vi "Periodic Tasks.vi"(8 "error in":errorcluster) -> ()   [LabVIEW 2019]
doc: "This VI runs in parallel to other tasks. It can contain as many user-defined periodic loops as you need. These can carry out PID or other sorts of timed response."
uses:
  <vilib>/Rock Robotics/WPI/DriverStation/WPI_DriverStationRobotMode2.ctl
  LabVIEW_is_Under_Control.lib/Util/Toggle/Change Detect.vi
  LabVIEW_is_Under_Control.lib/Util/Toggle/Change Detect Boolean.vi
  <vilib>/Rock Robotics/WPI/Utilities/WPI_GetSetVariantRefNum.vi
  Robot Global Data.vi
  StateMachine_Global.vi
  Axes_n_Buttons_Global.vi
  Actuators_n_Sensor_Global.vi
  <vilib>/Rock Robotics/WPI/ThirdParty/Phoenix-LabVIEW/Motor Controller/Controls/CTRE_Phoenix_MotorControl_ControlMode.ctl
  <vilib>/Rock Robotics/WPI/Solenoid/WPI_SolenoidValue.ctl
  <vilib>/Rock Robotics/WPI/Solenoid/WPI_SolenoidSetEnum.vi
  <vilib>/Rock Robotics/Network Tables/NT Read Number.vi
  <vilib>/Rock Robotics/Network Tables/NT Write Number.vi
  StateMachines/Turret_Control.ctl
  StateMachines/Climber_Control.ctl
  <vilib>/Rock Robotics/WPI/ThirdParty/Phoenix-LabVIEW/Motor Controller/Controls/CTRE_Phoenix_MotorControl_FeedbackDevice.ctl
  <vilib>/Rock Robotics/WPI/ThirdParty/Phoenix-LabVIEW/Motor Controller/Get/CTRE_Phoenix_MotorController_GetSelectedSensorData.vi
  <vilib>/Rock Robotics/WPI/ThirdParty/Phoenix-LabVIEW/Motor Controller/Get/CTRE_Phoenix_MotorController_GetVoltage.vi
  StateMachines/Ball_Control.ctl
panel:
  in  "Corsair Control":T1(tab)=enum."Turret"
  out "Right Current":dbl
  out "Left Current":dbl
  out "Reversed?":bool
  out "Left Side Current":cluster{"current (A)":dbl, "current (A)":dbl}(graph)
  in  "Sensitivity":dbl=1.5
  out "Right Side Current":cluster{"current (A)":dbl, "current (A)":dbl}(graph)
  out "Voltage Chart":cluster{"Percent Output":dbl}(graph)
  in  "I Zone":dbl
  in  "kF":dbl
  in  "D":dbl
  in  "I":dbl
  in  "P":dbl
  in  "Neutral to Full Seconds":dbl=0.2
  out "Shooter PID Chart":cluster{"Shooter Setpoint":dbl, dbl}(graph)
  out "Voltage Chart Hood":cluster{"Percent Output":dbl}(graph)
  out "Shooter PID Chart Hood":cluster{"Shooter Setpoint":dbl, dbl}(graph)
  in  "I Zone Hood":dbl
  in  "kF Hood":dbl
  in  "D Hood":dbl
  in  "I Hood":dbl
  in  "P Hood":dbl
  in  "Neutral to Full Seconds Hood":dbl=0.2
  out "Turret PID Chart":cluster{"Turret Setpoint":dbl, "TAoutput":dbl}(graph)
  in  "TARange":cluster{"output high":dbl, "output low":dbl}={"output high"=0.6, "output low"=-0.6} {"output low" format="%.2f"; "output high" format="%.2f"}
  in  "TAIntegral Range":dbl=10000.0
  in  "TADisable Range":dbl
  in  "TAGains":T2={"proportional gain (Kc)"=1.0, "integral time (Ti, min)"=0.01, "derivative time (Td, min)"=0.0} {"derivative time (Td, min)" format="%.3f"; "integral time (Ti, min)" format="%.3f"; "proportional gain (Kc)" format="%.3f"}
  out "Hood PID Chart":cluster{"Turret Setpoint":dbl, "TAoutput":dbl}(graph)
  in  "HGains":T2={"proportional gain (Kc)"=1.0, "integral time (Ti, min)"=0.01, "derivative time (Td, min)"=0.0} {"derivative time (Td, min)" format="%.3f"; "integral time (Ti, min)" format="%.3f"; "proportional gain (Kc)" format="%.3f"}
  in  "HDisable Range":dbl
  in  "HIntegral Range":dbl=10000.0
  in  "HRange":cluster{"output high":dbl, "output low":dbl}={"output high"=0.6, "output low"=-0.6} {"output low" format="%.2f"; "output high" format="%.2f"}
  in  "Climber Setpoint":dbl
  in  "Climber Output":dbl
  in  "PDP Port":i32
  out "Current":dbl
  out "Pressing?":bool
  in  "Debug %":dbl
  out "Debug Current":cluster{"current (A)":dbl}(graph)
  # "Press USB 0 A button"
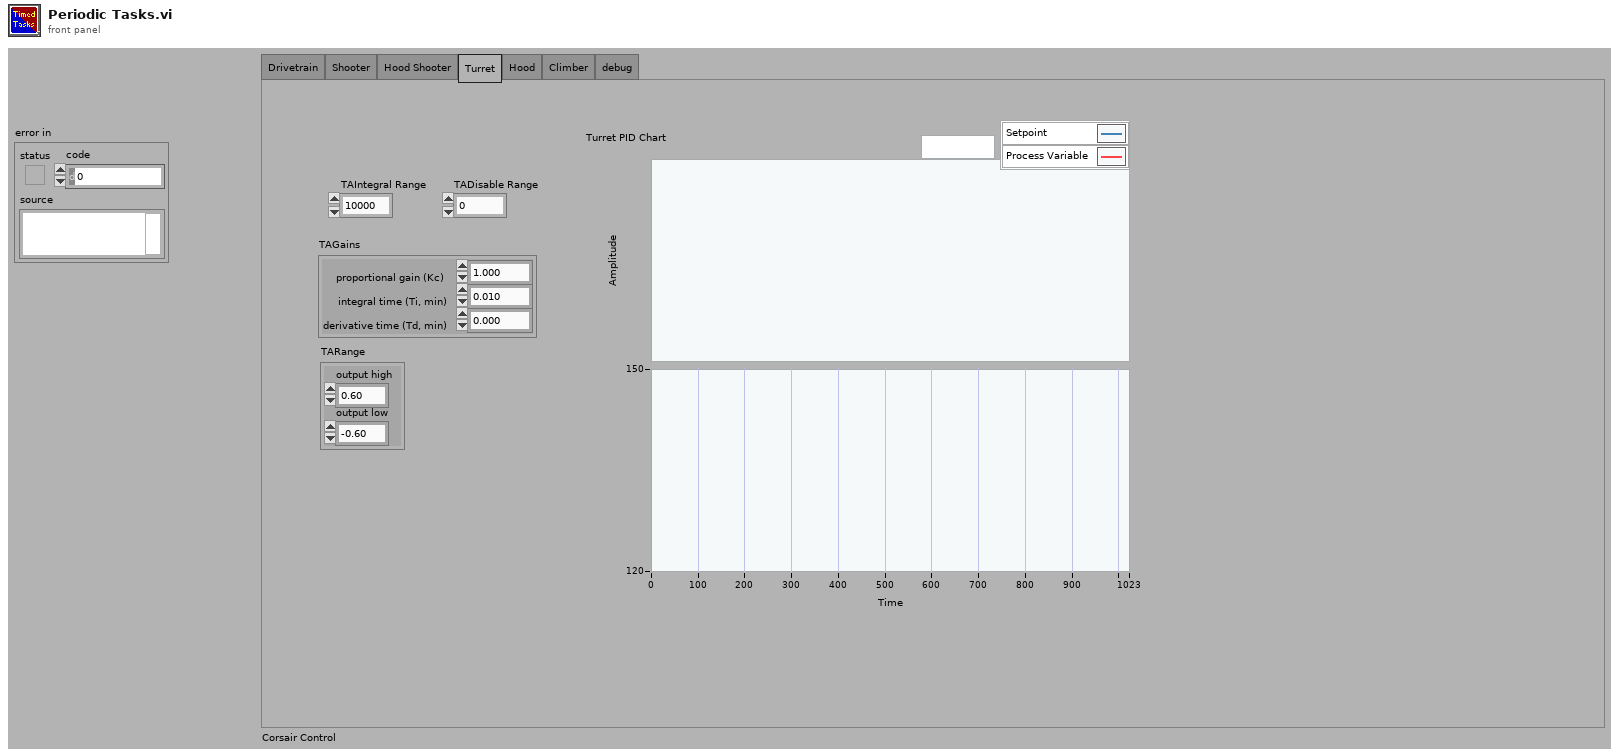
[diagram p1: front panel]
types:
  T1 = enum32{"Drivetrain", "Shooter", "Hood Shooter", "Turret", "Hood", "Climber", "debug"}
  T2 = cluster{"proportional gain (Kc)":dbl, "integral time (Ti, min)":dbl, "derivative time (Td, min)":dbl}
  T3 = typedef "WPI_MotorControlDeviceRef.ctl" = cluster{"DeviceStatus":errorcluster, "Type":T4, "PWM":cluster{"PWM Channel":T5, "DeadBand":T6}, "CAN":cluster{"Device Number":u8, "SetOutput VI Ref":variant, "GetOutput VI Ref":variant, "Enable VI Ref":variant, "Disable VI Ref":variant, "Data":variant}, "Invert":bool, "DIO PWM":cluster{"PWM \"Enable\" Channel":T5, "DIOChannel":T7, "PWM Rate":dbl}}
  T4 = typedef "WPI_MotorControlType.ctl" = enum16{"PWM", "CAN", "DIO PWM"}
  T5 = typedef "FPGA_DIOPWMChannel.ctl" = enum8{"PWM 0", "PWM 1", "PWM 2", "PWM 3", "PWM 4", "PWM 5", "PWM 6", "PWM 7", "PWM 8", "PWM 9", "PWM MXP 0", "PWM MXP 1", "PWM MXP 2", "PWM MXP 3", "PWM MXP 4", "PWM MXP 5", "PWM MXP 6", "PWM MXP 7", "PWM MXP 8", "PWM MXP 9", "Invalid"}
  T6 = typedef "WPI_PWMDeadband.ctl" = cluster{"Name":string, "maxPositivePwm":i32, "minPositivePwm":i32, "centerPwm":i32, "maxNegativePwm":i32, "minNegativePwm":i32, "angularRange":u16}
  T7 = typedef "FPGA_DIOChannel.ctl" = enum8{"DIO 0", "DIO 1", "DIO 2", "DIO 3", "DIO 4", "DIO 5", "DIO 6", "DIO 7", "DIO 8", "DIO 9", "DIO MXP 0", "DIO MXP 1", "DIO MXP 2", "DIO MXP 3", "DIO MXP 4", "DIO MXP 5", "DIO MXP 6", "DIO MXP 7", "DIO MXP 8", "DIO MXP 9", "DIO MXP 10", "DIO MXP 11", "DIO MXP 12", "DIO MXP 13", "DIO MXP 14", "DIO MXP 15", "SPI Port CS1", "SPI Port CS2", "SPI Port CS3", "SPI Port MISO", "SPI Port MOSI", "Invalid"}
  T8 = typedef "WPI_SolenoidDevRef.ctl" = cluster{"DevStatus":errorcluster, "Pneumatics Control Module":u8, "Forward Solenoid Channel":T9, "Reverse Solenoid Channel":T9}
  T9 = typedef "WPI_SolenoidChannel.ctl" = enum8{"Solenoid 0", "Solenoid 1", "Solenoid 2", "Solenoid 3", "Solenoid 4", "Solenoid 5", "Solenoid 6", "Solenoid 7", "Invalid"}
  T10 = typedef "WPI_EncoderDevRef.ctl" = cluster{"DevStatus":errorcluster, "EncoderIndex":T11, "CounterIndex":T12, "DistancePerCount":dbl, "Decoding Type":T13}
  T11 = typedef "FPGA_EncoderIdx.ctl" = enum8{"Enc 0", "Enc 1", "Enc 2", "Enc 3", "Enc 4", "Enc 5", "Enc 6", "Enc 7", "Invalid"}
  T12 = typedef "FPGA_CounterCtrSystemIndex.ctl" = enum8{"Ctr 0", "Ctr 1", "Ctr 2", "Ctr 3", "Ctr 4", "Ctr 5", "Ctr 6", "Ctr 7", "Invalid"}
  T13 = typedef "WPI_EncoderType.ctl" = enum16{"1x", "2x", "4x"}
  T14 = typedef "WPI_RobotDriveDevRef.ctl" = cluster{"DevStatus":errorcluster, "Motors[]":T3[], "Square Inputs":bool, "Max Output":dbl}
  T15 = typedef "WPI_JoystickDevRef.ctl" = cluster{"Device":T16}
  T16 = typedef "WPI_JoystickDeviceEnum.ctl" = enum16{"USB 0", "USB 1", "USB 2", "USB 3", "USB 4", "USB 5"}
  T17 = typedef "WPI_SolenoidValue.ctl" = enum16{"Off", "On", "Forward", "Reverse"}
  T18 = typedef "CTRE_Phoenix_MotorControl_ControlMode.ctl" = u16
  T19 = cluster{"Motors[][0]":T3, "Motors[][1]":T3, "Motors[][2]":T3, "Motors[][3]":T3, "Motors[][4]":T3, "Motors[][5]":T3, "Motors[][6]":T3, "Motors[][7]":T3, "Motors[][8]":T3}
  T20 = typedef "Ball_Control.ctl" = enum16{"Default", "Collect Power Cells", "Prepare Shooter", "Shoot", "Climber Lock"}
  T21 = typedef "Climber_Control.ctl" = enum16{"Locked", "Extend", "Aligned", "Pull", "Lock PTO"}
  T22 = typedef "Turret_Control.ctl" = enum16{"Static", "PreDefined", "Limelight", "Free Control", "Dragoon Mode"}
  T23 = typedef "CTRE_Phoenix_MotorControl_FeedbackDevice.ctl" = i8
  T24 = typedef "WPI_DriverStationRobotMode2.ctl" = enum16{"Autonomous Disabled", "Autonomous Enabled", "Teleop Disabled", "Teleop Enabled", "Disconnected", "Finish", "Test Disabled", "Test Enabled", "Emergency Stopped"}
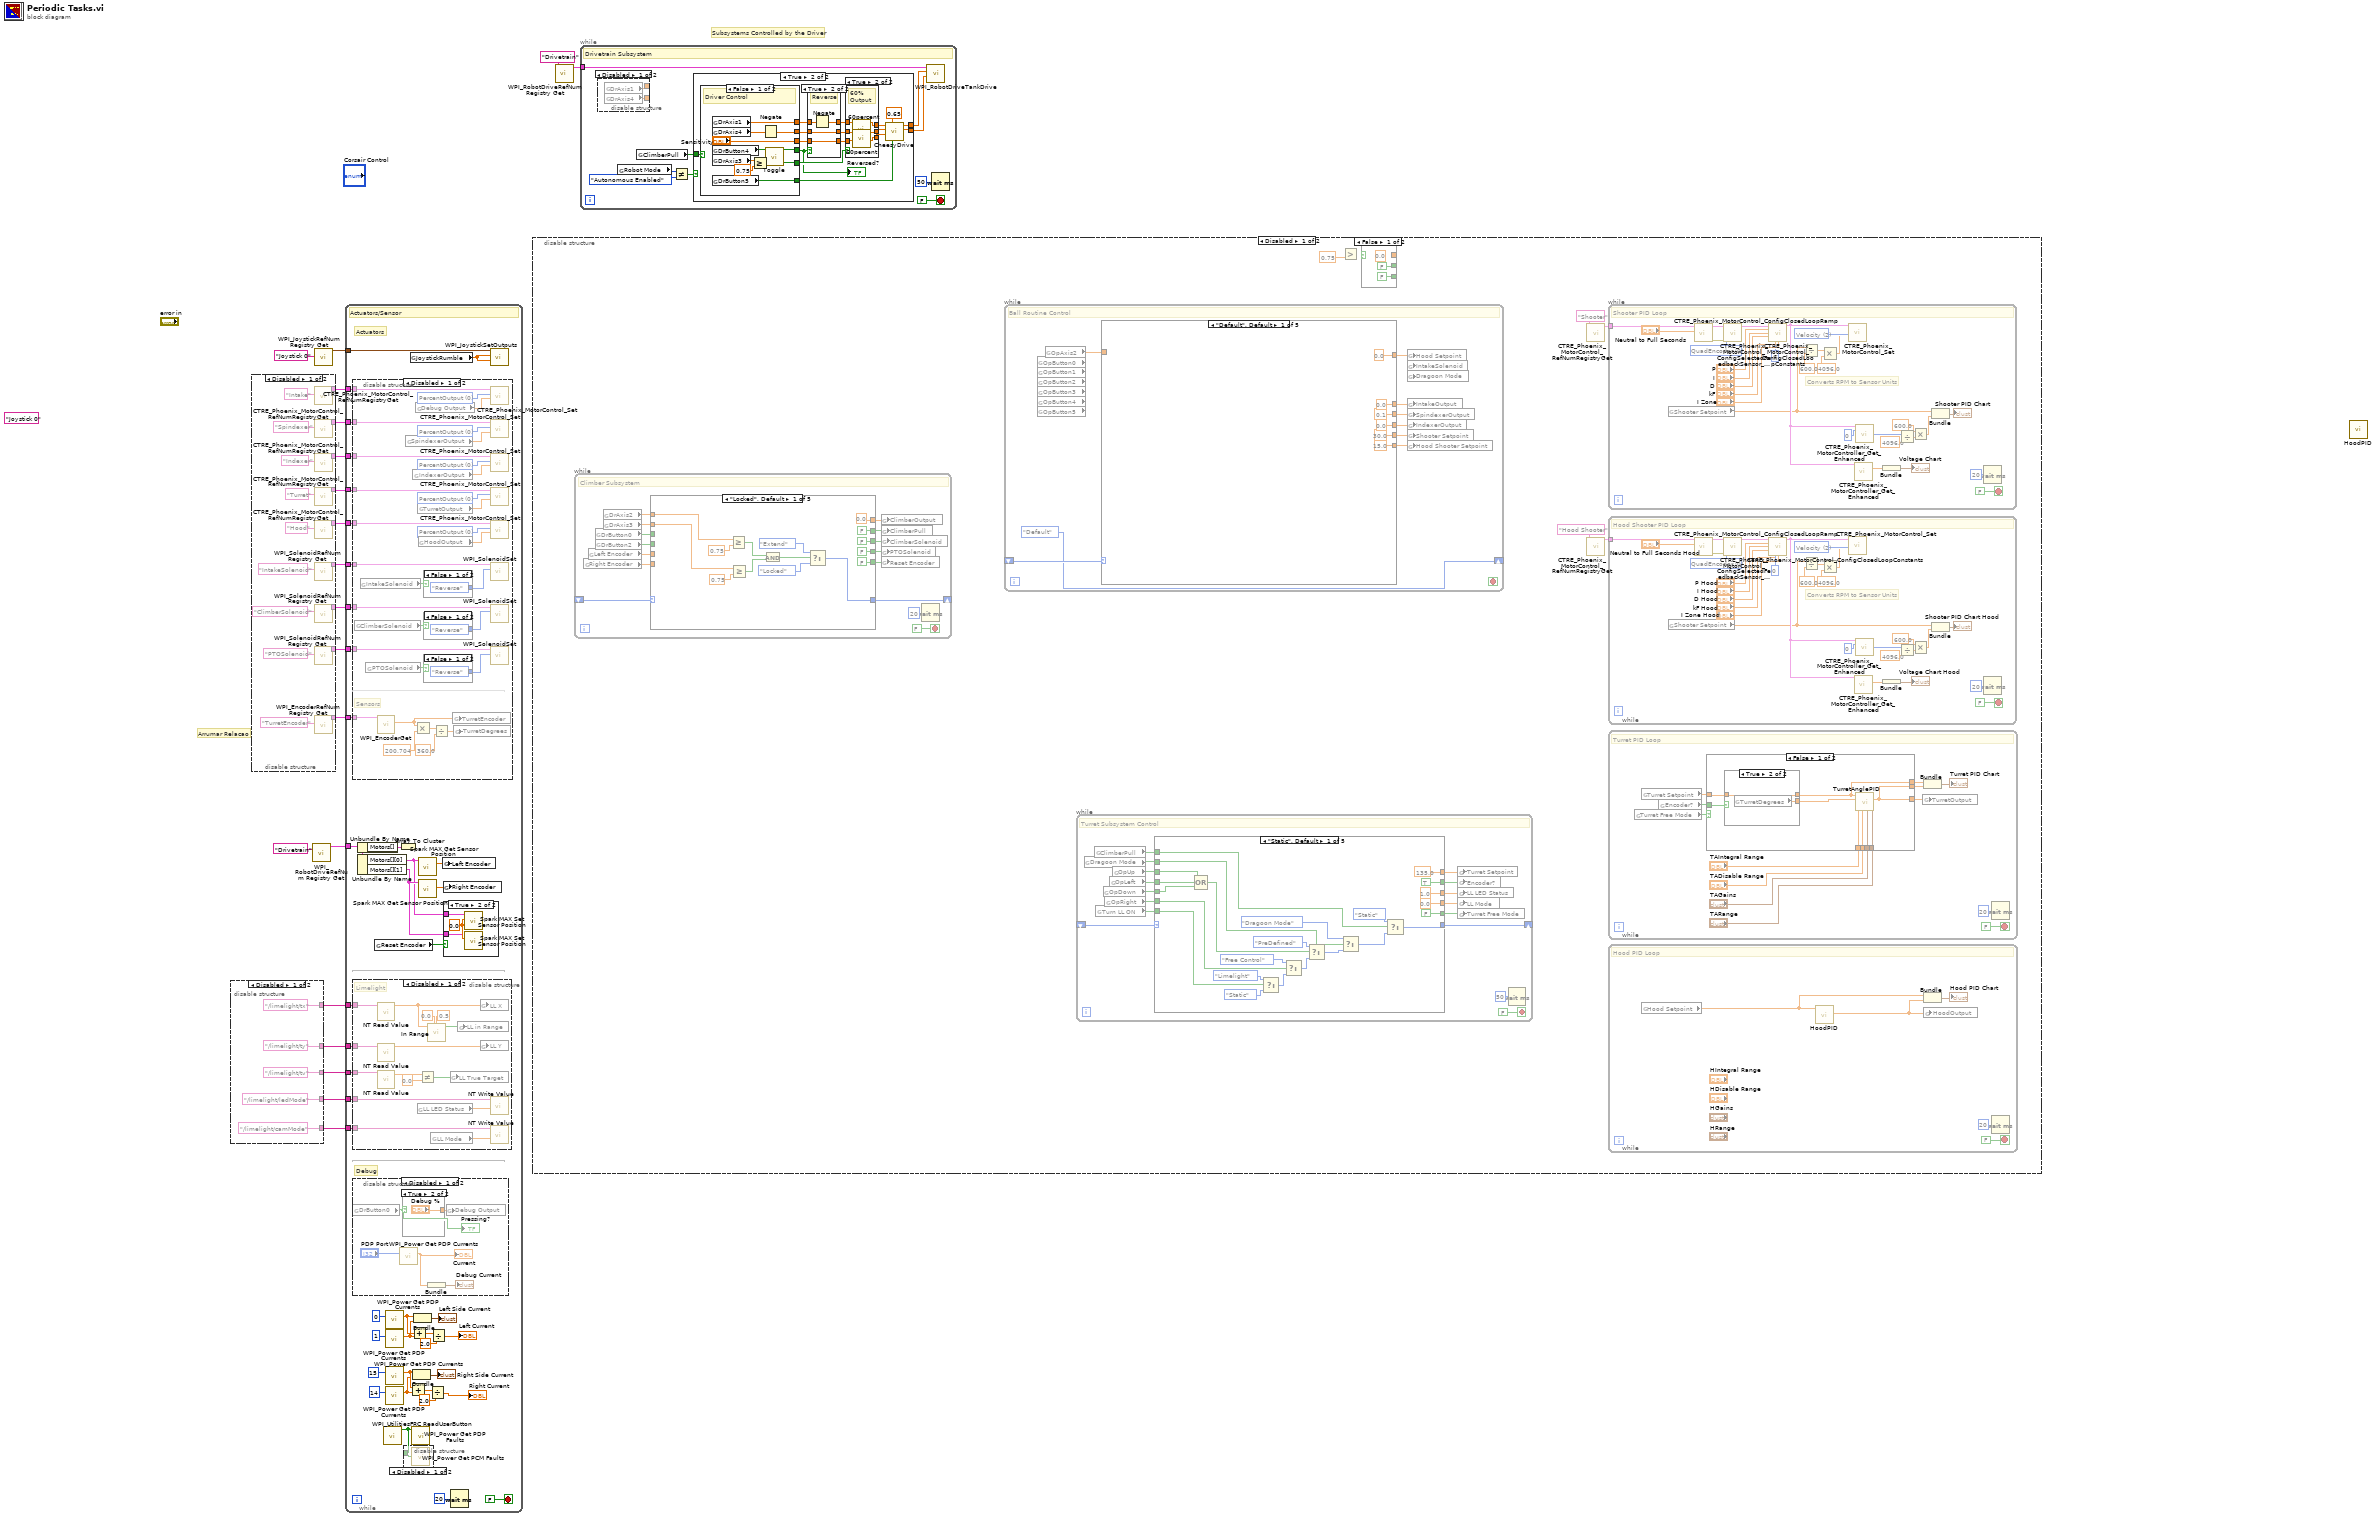
[diagram p0: block diagram]
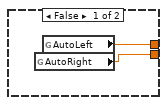
[diagram p3: hidden frame]
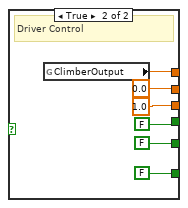
[diagram p5: hidden frame]
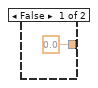
[diagram p9: hidden frame]
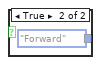
[diagram p13: hidden frame]
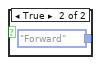
[diagram p14: hidden frame]
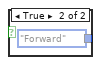
[diagram p15: hidden frame]
diagram:
  (unwired) "Joystick 0" ("refnum name")
  # "Subsystems Controlled by the Driver"
  # "Arrumar Relacao"
  n1 = disable-structure shown="Disabled" {
    disable-tunnel: ["/limelight/tx" ("Name") _] -> w13
    disable-tunnel: ["/limelight/ty" ("Name") _] -> w12
    disable-tunnel: ["/limelight/tv" ("Name") _] -> w11
    disable-tunnel: ["/limelight/ledMode" ("Name") _] -> w10
    disable-tunnel: ["/limelight/camMode" ("Name") _] -> w9
    frame Disabled {
    }
    frame Enabled {
    }
  }
  n2 = disable-structure shown="Disabled" {
    disable-tunnel: [w42 _] -> w20
    disable-tunnel: [w41 _] -> w19
    disable-tunnel: [w38 _] -> w18
    disable-tunnel: [w37 _] -> w17
    disable-tunnel: [w34 _] -> w16
    disable-tunnel: [w33 _] -> w15
    disable-tunnel: [w32 _] -> w7
    disable-tunnel: [w31 _] -> w6
    disable-tunnel: [w30 _] -> w5
    frame Disabled {
      n3 = call <vilib>:"CTRE_Phoenix_MotorControl_RefNumRegistryGet.vi"("refnum name"="Intake") -> ("PhoenixMotorControlDevRef"=w42:T3)  [unwired: 9 in, 1 out]
      n4 = call <vilib>:"CTRE_Phoenix_MotorControl_RefNumRegistryGet.vi"("refnum name"="Spindexer") -> ("PhoenixMotorControlDevRef"=w41:T3)  [unwired: 9 in, 1 out]
      n5 = call <vilib>:"CTRE_Phoenix_MotorControl_RefNumRegistryGet.vi"("refnum name"="Indexer") -> ("PhoenixMotorControlDevRef"=w38:T3)  [unwired: 9 in, 1 out]
      n6 = call <vilib>:"CTRE_Phoenix_MotorControl_RefNumRegistryGet.vi"("refnum name"="Turret") -> ("PhoenixMotorControlDevRef"=w37:T3)  [unwired: 9 in, 1 out]
      n7 = call <vilib>:"CTRE_Phoenix_MotorControl_RefNumRegistryGet.vi"("refnum name"="Hood") -> ("PhoenixMotorControlDevRef"=w34:T3)  [unwired: 9 in, 1 out]
      n8 = call <vilib>:"WPI_SolenoidRefNum Registry Get.vi"("refnum name"="IntakeSolenoid") -> ("SolenoidDevRef"=w32:T8)  [unwired: 9 in, 1 out]
      n9 = call <vilib>:"WPI_SolenoidRefNum Registry Get.vi"("refnum name"="ClimberSolenoid") -> ("SolenoidDevRef"=w31:T8)  [unwired: 9 in, 1 out]
      n10 = call <vilib>:"WPI_SolenoidRefNum Registry Get.vi"("refnum name"="PTOSolenoid") -> ("SolenoidDevRef"=w30:T8)  [unwired: 9 in, 1 out]
      n11 = call <vilib>:"WPI_EncoderRefNum Registry Get.vi"("refnum name"="TurretEncoder") -> ("EncoderDevRef"=w33:T10)  [unwired: 9 in, 1 out]
    }
    frame Enabled {
    }
  }
  n12 = call <vilib>:"WPI_RobotDriveRefNum Registry Get.vi"("refnum name"="Drivetrain") -> ("RobotDriveDevRef"=w3:T14)  [unwired: 9 in, 1 out]
  n13 = call <vilib>:"WPI_JoystickRefNum Registry Get.vi"("refnum name"="Joystick 0") -> ("JoystickDevRef"=w14:T15)  [unwired: 9 in, 1 out]
  n14 = while {
    tunnel: w20 -> [w86]
    tunnel: w19 -> [w85]
    tunnel: w18 -> [w84]
    tunnel: w17 -> [w83]
    tunnel: w16 -> [w82]
    tunnel: w15 -> [w81]
    tunnel: w14 -> [w80]
    tunnel: w13 -> [w78]
    tunnel: w12 -> [w77]
    tunnel: w11 -> [w76]
    tunnel: w10 -> [w75]
    tunnel: w9 -> [w74]
    tunnel: w7 -> [w72]
    tunnel: w6 -> [w71]
    tunnel: w5 -> [w70]
    tunnel: w3 -> [w69]
    stop <- FALSE stop-if-true
    # "Debug"
    # "Actuators"
    # "Actuators/Sensor"
    n15 = disable-structure shown="Disabled" {
      disable-tunnel: w86 -> [w139 _]
      disable-tunnel: w85 -> [w138 _]
      disable-tunnel: w84 -> [w137 _]
      disable-tunnel: w83 -> [w136 _]
      disable-tunnel: w82 -> [w135 _]
      disable-tunnel: w81 -> [w128 _]
      disable-tunnel: w72 -> [w117 _]
      disable-tunnel: w71 -> [w116 _]
      disable-tunnel: w70 -> [w115 _]
      frame Disabled {
        w126 = T18 0 items=["PercentOutput"=0, "Position"=1, "Velocity"=2, "Current"=3, "Follower"=5, "MotionProfile"=6, "MotionMagic"=7, "MotionProfileArc"=10, "Disabled"=15] ("Control Mode")
        w121 = T18 0 items=["PercentOutput"=0, "Position"=1, "Velocity"=2, "Current"=3, "Follower"=5, "MotionProfile"=6, "MotionMagic"=7, "MotionProfileArc"=10, "Disabled"=15] ("Control Mode")
        w123 = T18 0 items=["PercentOutput"=0, "Position"=1, "Velocity"=2, "Current"=3, "Follower"=5, "MotionProfile"=6, "MotionMagic"=7, "MotionProfileArc"=10, "Disabled"=15] ("Control Mode")
        w125 = T18 0 items=["PercentOutput"=0, "Position"=1, "Velocity"=2, "Current"=3, "Follower"=5, "MotionProfile"=6, "MotionMagic"=7, "MotionProfileArc"=10, "Disabled"=15] ("Control Mode")
        w127 = T18 0 items=["PercentOutput"=0, "Position"=1, "Velocity"=2, "Current"=3, "Follower"=5, "MotionProfile"=6, "MotionMagic"=7, "MotionProfileArc"=10, "Disabled"=15] ("Control Mode")
        # "Sensors"
        n16 = global read "Actuators_n_Sensor_Global.vi" "ClimberSolenoid"() -> (w132:bool)
        n17 = global read "Actuators_n_Sensor_Global.vi" "IntakeSolenoid"() -> (w133:bool)
        n18 = global read "Actuators_n_Sensor_Global.vi" "PTOSolenoid"() -> (w129:bool)
        n19 = call <vilib>:"WPI_EncoderGet.vi"("EncoderDevRef"=w128) -> ("Distance"=w110:dbl)  [unwired: 5 in, 5 out]
        n20 = global read "Actuators_n_Sensor_Global.vi" "SpindexerOutput"() -> (w124:dbl)
        n21 = global read "Actuators_n_Sensor_Global.vi" "IndexerOutput"() -> (w122:dbl)
        n22 = Multiply(x=w110, y=200.704) -> (x*y=w113:dbl)
        n23 = global read "Actuators_n_Sensor_Global.vi" "Debug Output"() -> (w118:dbl)
        n24 = global read "Actuators_n_Sensor_Global.vi" "TurretOutput"() -> (w120:dbl)
        n25 = global read "Actuators_n_Sensor_Global.vi" "HoodOutput"() -> (w119:dbl)
        n26 = case shown="False" w133 {
          tunnel: [WPI_SolenoidValue."Reverse" ("Value") WPI_SolenoidValue."Forward" ("Value")] -> w134
          frame False {
          }
          frame True {
          }
        }
        n27 = case shown="False" w132 {
          tunnel: [WPI_SolenoidValue."Reverse" ("Value") WPI_SolenoidValue."Forward" ("Value")] -> w131
          frame False {
          }
          frame True {
          }
        }
        n28 = case shown="False" w129 {
          tunnel: [WPI_SolenoidValue."Reverse" ("Value") WPI_SolenoidValue."Forward" ("Value")] -> w130
          frame False {
          }
          frame True {
          }
        }
        n29 = Divide(x=w113, y=360.0) -> (x/y=w111:dbl)
        n30 = global write "Actuators_n_Sensor_Global.vi" "TurretEncoder"(w110) -> ()
        n31 = global write "Actuators_n_Sensor_Global.vi" "TurretDegrees"(w111) -> ()
        n32 = call <vilib>:"CTRE_Phoenix_MotorControl_Set.vi"("Output"=w118, "Control Mode"=w127, "PhoenixMotorControlDevRef"=w139) -> ()  [unwired: 7 in, 2 out]
        n33 = call <vilib>:"CTRE_Phoenix_MotorControl_Set.vi"("Output"=w124, "Control Mode"=w125, "PhoenixMotorControlDevRef"=w138) -> ()  [unwired: 7 in, 2 out]
        n34 = call <vilib>:"CTRE_Phoenix_MotorControl_Set.vi"("Output"=w122, "Control Mode"=w123, "PhoenixMotorControlDevRef"=w137) -> ()  [unwired: 7 in, 2 out]
        n35 = call <vilib>:"CTRE_Phoenix_MotorControl_Set.vi"("Output"=w120, "Control Mode"=w121, "PhoenixMotorControlDevRef"=w136) -> ()  [unwired: 7 in, 2 out]
        n36 = call <vilib>:"CTRE_Phoenix_MotorControl_Set.vi"("Output"=w119, "Control Mode"=w126, "PhoenixMotorControlDevRef"=w135) -> ()  [unwired: 7 in, 2 out]
        n37 = call-poly <vilib>:"WPI_SolenoidSet.vi"("Value"=w134, "SolenoidDevRef"=w117) -> ()  [unwired: 8 in, 2 out]
        n38 = call-poly <vilib>:"WPI_SolenoidSet.vi"("Value"=w131, "SolenoidDevRef"=w116) -> ()  [unwired: 8 in, 2 out]
        n39 = call-poly <vilib>:"WPI_SolenoidSet.vi"("Value"=w130, "SolenoidDevRef"=w115) -> ()  [unwired: 8 in, 2 out]
      }
      frame Enabled {
      }
    }
    n40 = disable-structure shown="Disabled" {
      frame Disabled {
        n41 = global read "Axes_n_Buttons_Global.vi" "DrButton0"() -> (w88:bool)
        "Pressing?" <- w88
        n42 = call <vilib>:"WPI_Power Get PDP Currents.vi"("PDP Channel"="PDP Port") -> ("current (A)"=w87:dbl)  [unwired: 12 in, 2 out]
        "Current" <- w87
        n43 = case shown="True" w88 {
          tunnel: [0.0 ("Test") "Debug %"] -> w91
          frame False {
          }
          frame True {
          }
        }
        n44 = Bundle("current (A)"=w87) -> (→"Debug Current":cluster{"current (A)":dbl})  [unwired: 1 in]
        n45 = global write "Actuators_n_Sensor_Global.vi" "Debug Output"(w91) -> ()
      }
      frame Enabled {
      }
    }
    n46 = disable-structure shown="Disabled" {
      disable-tunnel: w78 -> [w101 _]
      disable-tunnel: w77 -> [w100 _]
      disable-tunnel: w76 -> [w99 _]
      disable-tunnel: w75 -> [w98 _]
      disable-tunnel: w74 -> [w97 _]
      frame Disabled {
        # "Limelight"
        n47 = call-poly <vilib>:"NT Read Value.vi"("Name"=w101) -> ("Numeric"=w108:dbl)  [unwired: 9 in, 1 out]
        n48 = call-poly <vilib>:"NT Read Value.vi"("Name"=w100) -> ("Numeric"=w105:dbl)  [unwired: 9 in, 1 out]
        n49 = call-poly <vilib>:"NT Read Value.vi"("Name"=w99) -> ("Numeric"=w103:dbl)  [unwired: 9 in, 1 out]
        n50 = global read "Actuators_n_Sensor_Global.vi" "LL LED Status"() -> (w96:dbl)
        n51 = Not Equal?(x=w103, y=0.0) -> (x != y?=w102:bool)
        n52 = call "In Range.vi"("Range"=0.5, "Setpoint"=0.0, "Value"=w108) -> ("in range?"=w109:bool)  [unwired: 8 in]
        n53 = global read "Actuators_n_Sensor_Global.vi" "LL Mode"() -> (w95:dbl)
        n54 = global write "Actuators_n_Sensor_Global.vi" "LL True Target"(w102) -> ()
        n55 = global write "Actuators_n_Sensor_Global.vi" "LL in Range"(w109) -> ()
        n56 = global write "Actuators_n_Sensor_Global.vi" "LL X"(w108) -> ()
        n57 = global write "Actuators_n_Sensor_Global.vi" "LL Y"(w105) -> ()
        n58 = call-poly <vilib>:"NT Write Value.vi"("Numeric"=w96, "Name"=w98) -> ()  [unwired: 9 in, 1 out]
        n59 = call-poly <vilib>:"NT Write Value.vi"("Numeric"=w95, "Name"=w97) -> ()  [unwired: 9 in, 1 out]
      }
      frame Enabled {
      }
    }
    n60 = Unbundle By Name(w69) -> ("Motors[]"=w68:T3[])
    n61 = global read "Actuators_n_Sensor_Global.vi" "Reset Encoder"() -> (w64:bool)
    n62 = call <vilib>:"WPI_UtilitiesFRC ReadUserButton.vi"() -> ("User Button"=w60:bool)  [unwired: 10 in, 1 out]
    n63 = call <vilib>:"WPI_Power Get PDP Currents.vi"("PDP Channel"=0) -> ("current (A)"=w53:dbl)  [unwired: 12 in, 2 out]
    n64 = call <vilib>:"WPI_Power Get PDP Currents.vi"("PDP Channel"=1) -> ("current (A)"=w52:dbl)  [unwired: 12 in, 2 out]
    n65 = call <vilib>:"WPI_Power Get PDP Currents.vi"("PDP Channel"=15) -> ("current (A)"=w46:dbl)  [unwired: 12 in, 2 out]
    n66 = call <vilib>:"WPI_Power Get PDP Currents.vi"("PDP Channel"=14) -> ("current (A)"=w45:dbl)  [unwired: 12 in, 2 out]
    n67 = Array To Cluster(array=w68) -> (cluster=w67:T19)
    n68 = Unbundle By Name(w67) -> ("Motors[][0]"=w62:T3, "Motors[][1]"=w63:T3)
    n69 = disable-structure shown="Disabled" {
      disable-tunnel: w60 -> [w94 _]
      frame Disabled {
        n70 = call <vilib>:"WPI_Power Get PCM Faults.vi"("Clear Sticky Faults"=w94) -> ()  [unwired: 11 in, 4 out]
      }
      frame Enabled {
      }
    }
    n71 = Add(x=w46, y=w45) -> (x+y=w47:dbl)
    n72 = global read "Actuators_n_Sensor_Global.vi" "JoystickRumble"() -> (w79:dbl)
    n73 = Add(x=w53, y=w52) -> (x+y=w51:dbl)
    n74 = call <vilib>:"WPI_Power Get PDP Faults.vi"("Clear Sticky Faults"=w60) -> ()  [unwired: 10 in, 5 out]
    n75 = Bundle("current (A)"=w46, "current (A)"=w45) -> (→"Right Side Current":cluster{"current (A)":dbl, "current (A)":dbl})  [unwired: 1 in]
    n76 = Bundle("current (A)"=w53, "current (A)"=w52) -> (→"Left Side Current":cluster{"current (A)":dbl, "current (A)":dbl})  [unwired: 1 in]
    n77 = call <vilib>:"Spark MAX Get Sensor Position.vi"("MotorControlDevRef in"=w62) -> ("Sensor Position"=w66:dbl)  [unwired: 7 in, 3 out]
    n78 = call <vilib>:"Spark MAX Get Sensor Position.vi"("MotorControlDevRef in"=w63) -> ("Sensor Position"=w65:dbl)  [unwired: 7 in, 3 out]
    n79 = Divide(x=w47, y=2.0) -> (x/y=→"Right Current":dbl)
    n80 = Divide(x=w51, y=2.0) -> (x/y=→"Left Current":dbl)
    n81 = global write "Actuators_n_Sensor_Global.vi" "Left Encoder"(w66) -> ()
    n82 = global write "Actuators_n_Sensor_Global.vi" "Right Encoder"(w65) -> ()
    n83 = case shown="True" w64 {
      tunnel: w63 -> [_ w147]
      tunnel: w62 -> [_ w146]
      frame False {
      }
      frame True {
        w148 = 0.0 ("Position")
        n84 = call <vilib>:"Spark MAX Set Sensor Position.vi"("Position"=w148, "MotorControlDeviceRef"=w146) -> ()  [unwired: 8 in, 2 out]
        n85 = call <vilib>:"Spark MAX Set Sensor Position.vi"("Position"=w148, "MotorControlDeviceRef"=w147) -> ()  [unwired: 8 in, 2 out]
      }
    }
    n86 = Wait (ms)(milliseconds to wait=u32 20) -> ()  [unwired: 1 out]
    n87 = call <vilib>:"WPI_JoystickSetOutputs.vi"("Right Rumble"=w79, "Left Rumble"=w79, "JoystickDevRef"=w80) -> ()  [unwired: 7 in, 2 out]
  }
  n88 = disable-structure shown="Disabled" {
    frame Disabled {
      n89 = while {
        shift-right: [w245] -> _
        shift-left: _ -> [w246]
        stop <- FALSE stop-if-true
        # "Climber Subsystem"
        n90 = global read "Actuators_n_Sensor_Global.vi" "Right Encoder"() -> (w239:dbl)
        n91 = global read "Actuators_n_Sensor_Global.vi" "Left Encoder"() -> (w240:dbl)
        n92 = global read "Axes_n_Buttons_Global.vi" "DrButton0"() -> (w242:bool)
        n93 = global read "Axes_n_Buttons_Global.vi" "DrButton2"() -> (w241:bool)
        n94 = global read "Axes_n_Buttons_Global.vi" "DrAxis2"() -> (w244:dbl)
        n95 = global read "Axes_n_Buttons_Global.vi" "DrAxis3"() -> (w243:dbl)
        n96 = case shown="\"Locked\", Default" w246 {
          tunnel: [w257 w265 Climber_Control."Pull" w282 Climber_Control."Lock PTO"] -> w245
          tunnel: w244 -> [w255 _ _ _ _]
          tunnel: w243 -> [w254 _ _ _ _]
          tunnel: w242 -> [_ w266 _ _ _]
          tunnel: w241 -> [_ _ _ _ _]
          tunnel: w240 -> [_ _ _ w292 _]
          tunnel: w239 -> [_ _ _ w293 _]
          tunnel: [FALSE FALSE FALSE TRUE FALSE] -> w238
          tunnel: [0.0 0.0 0.0 "Climber Output" 0.0 ("Climber Output")] -> w237
          tunnel: [FALSE TRUE TRUE TRUE TRUE] -> w236
          tunnel: [FALSE FALSE TRUE TRUE FALSE] -> w235
          tunnel: [FALSE FALSE TRUE FALSE TRUE] -> w234
          frame "Locked", Default {
            n97 = Greater Or Equal?(x=w255, y=0.75) -> (x >= y?=w261:bool)
            n98 = Greater Or Equal?(x=w254, y=0.75) -> (x >= y?=w260:bool)
            n99 = And(x=w261, y=w260) -> (x .and. y?=w259:bool)
            n100 = Select(t=Climber_Control."Extend", s=w259, f=Climber_Control."Locked") -> (s? t:f=w257:T21)
          }
          frame "Extend" {
            n101 = Select(t=Climber_Control."Aligned", s=w266, f=Climber_Control."Extend") -> (s? t:f=w265:T21)
          }
          frame "Aligned" {
          }
          frame "Pull" {
            n102 = Add(x=w292, y=w293) -> (x+y=w291:dbl)
            n103 = Divide(x=w291, y=2.0) -> (x/y=w289:dbl)
            n104 = Greater Or Equal?(x=w289, y="Climber Setpoint") -> (x >= y?=w283:bool)
            n105 = Select(t=Climber_Control."Lock PTO", s=w283, f=Climber_Control."Pull") -> (s? t:f=w282:T21)
          }
          frame "Lock PTO" {
          }
        }
        n106 = global write "StateMachine_Global.vi" "ClimberOutput"(w237) -> ()
        n107 = global write "StateMachine_Global.vi" "ClimberPull"(w238) -> ()
        n108 = global write "Actuators_n_Sensor_Global.vi" "ClimberSolenoid"(w236) -> ()
        n109 = global write "Actuators_n_Sensor_Global.vi" "PTOSolenoid"(w235) -> ()
        n110 = global write "Actuators_n_Sensor_Global.vi" "Reset Encoder"(w234) -> ()
        n111 = Wait (ms)(milliseconds to wait=u32 20) -> ()  [unwired: 1 out]
      }
      n112 = while {
        shift-right: [Ball_Control."Default"] -> _
        shift-left: _ -> [w167]
        stop <- _ stop-if-true
        # "Ball Routine Control"
        n113 = global read "Axes_n_Buttons_Global.vi" "OpButton0"() -> ()  [unwired: 1 out]
        n114 = global read "Axes_n_Buttons_Global.vi" "OpButton1"() -> ()  [unwired: 1 out]
        n115 = global read "Axes_n_Buttons_Global.vi" "OpButton2"() -> ()  [unwired: 1 out]
        n116 = global read "Axes_n_Buttons_Global.vi" "OpButton3"() -> ()  [unwired: 1 out]
        n117 = global read "Axes_n_Buttons_Global.vi" "OpButton4"() -> ()  [unwired: 1 out]
        n118 = global read "Axes_n_Buttons_Global.vi" "OpButton5"() -> ()  [unwired: 1 out]
        n119 = global read "Axes_n_Buttons_Global.vi" "OpAxis2"() -> (w160:dbl)
        n120 = case shown="\"Default\", Default" w167 {
          tunnel: [0.0 _ _ _ _] -> w165
          tunnel: [0.1 _ _ _ _] -> w164
          tunnel: [0.0 _ _ _ _] -> w163
          tunnel: [30.0 _ _ _ _] -> w162
          tunnel: [15.0 _ _ _ _] -> w161
          tunnel: w160 -> [_ _ _ _ _]
          tunnel: [0.0 _ _ _ _] -> w159
          frame "Default", Default {
          }
          frame "Collect Power Cells" {
          }
          frame "Prepare Shooter" {
          }
          frame "Shoot" {
          }
          frame "Climber Lock" {
          }
        }
        n121 = global write "StateMachine_Global.vi" "Hood Setpoint"(w159) -> ()
        n122 = global read "Actuators_n_Sensor_Global.vi" "IntakeSolenoid"() -> ()  [unwired: 1 in]
        n123 = global read "StateMachine_Global.vi" "Dragoon Mode"() -> ()  [unwired: 1 in]
        n124 = global write "Actuators_n_Sensor_Global.vi" "IntakeOutput"(w165) -> ()
        n125 = global write "Actuators_n_Sensor_Global.vi" "SpindexerOutput"(w164) -> ()
        n126 = global write "Actuators_n_Sensor_Global.vi" "IndexerOutput"(w163) -> ()
        n127 = global write "StateMachine_Global.vi" "Shooter Setpoint"(w162) -> ()
        n128 = global write "StateMachine_Global.vi" "Hood Shooter Setpoint"(w161) -> ()
      }
      n129 = while {
        shift-right: [w307] -> _
        shift-left: _ -> [w314]
        stop <- FALSE stop-if-true
        # "Turret Subsystem Control"
        n130 = global read "StateMachine_Global.vi" "Dragoon Mode"() -> (w303:bool)
        n131 = global read "StateMachine_Global.vi" "ClimberPull"() -> (w300:bool)
        n132 = global read "StateMachine_Global.vi" "Turn LL ON"() -> (w308:bool)
        n133 = global read "Axes_n_Buttons_Global.vi" "OpDown"() -> (w310:bool)
        n134 = global read "Axes_n_Buttons_Global.vi" "OpRight"() -> (w309:bool)
        n135 = global read "Axes_n_Buttons_Global.vi" "OpLeft"() -> (w311:bool)
        n136 = global read "Axes_n_Buttons_Global.vi" "OpUp"() -> (w312:bool)
        n137 = case shown="\"Static\", Default" w314 {
          tunnel: [135.0 w344 0.0 ("f") 0.0 ("f") 225.0 ("f")] -> w313
          tunnel: w312 -> [w338 w346 _ _ _]
          tunnel: w311 -> [w337 w347 _ _ _]
          tunnel: w310 -> [w336 w345 _ _ _]
          tunnel: w309 -> [w330 _ _ w364 _]
          tunnel: w308 -> [w329 _ w355 _ _]
          tunnel: [w319 w340 w356 w365 w375] -> w307
          tunnel: [0.0 _ _ _ _] -> w306
          tunnel: [1.0 1.0 0.0 1.0 1.0] -> w305
          tunnel: [TRUE TRUE FALSE FALSE TRUE] -> w304
          tunnel: w303 -> [w322 _ _ _ w374]
          tunnel: [FALSE _ _ TRUE _] -> w302
          tunnel: w300 -> [w316 _ _ _ _]
          frame "Static", Default {
            n138 = Compound Arithmetic op=OR(w338, w337, w336) -> (w335:bool)
            n139 = Select(t=Turret_Control."Limelight", s=w329, f=Turret_Control."Static") -> (s? t:f=w333:T22)
            n140 = Select(t=Turret_Control."Free Control", s=w330, f=w333) -> (s? t:f=w334:T22)
            n141 = Select(t=Turret_Control."PreDefined", s=w335, f=w334) -> (s? t:f=w323:T22)
            n142 = Select(t=Turret_Control."Dragoon Mode", s=w322, f=w323) -> (s? t:f=w318:T22)
            n143 = Select(t=Turret_Control."Static", s=w316, f=w318) -> (s? t:f=w319:T22)
          }
          frame "PreDefined" {
            n144 = Compound Arithmetic op=OR(w346, w347, w345) -> (w352:bool)
            n145 = Not(x=w352) -> (.not. x?=w349:bool)
            n146 = Select(t=225.0, s=w345, f=135.0) -> (s? t:f=w348:dbl)
            n147 = Select(t=45.0, s=w346, f=w348) -> (s? t:f=w344:dbl)
            n148 = Select(t=Turret_Control."Static", s=w349, f=Turret_Control."PreDefined") -> (s? t:f=w340:T22)
          }
          frame "Limelight" {
            n149 = Not(x=w355) -> (.not. x?=w358:bool)
            n150 = Select(t=Turret_Control."Static", s=w358, f=Turret_Control."Limelight") -> (s? t:f=w356:T22)
          }
          frame "Free Control" {
            n151 = Not(x=w364) -> (.not. x?=w363:bool)
            n152 = Select(t=Turret_Control."Static", s=w363, f=Turret_Control."PreDefined") -> (s? t:f=w365:T22)
          }
          frame "Dragoon Mode" {
            n153 = Not(x=w374) -> (.not. x?=w373:bool)
            n154 = Select(t=Turret_Control."Static", s=w373, f=Turret_Control."Dragoon Mode") -> (s? t:f=w375:T22)
          }
        }
        n155 = global write "StateMachine_Global.vi" "Turret Setpoint"(w313) -> ()
        n156 = global write "StateMachine_Global.vi" "Encoder?"(w304) -> ()
        n157 = global write "Actuators_n_Sensor_Global.vi" "LL LED Status"(w305) -> ()
        n158 = global write "Actuators_n_Sensor_Global.vi" "LL Mode"(w306) -> ()
        n159 = global write "StateMachine_Global.vi" "Turret Free Mode"(w302) -> ()
        n160 = Wait (ms)(milliseconds to wait=u32 50) -> ()  [unwired: 1 out]
      }
      n161 = Greater?(y=0.75) -> ()  [unwired: 1 in, 1 out]
      n162 = case shown="False" {
        selector: _ -> [_ _]
        tunnel: [FALSE TRUE] -> _
        tunnel: [FALSE TRUE] -> _
        tunnel: [_ 0.0] -> _
        frame False {
          (unwired) 0.0
        }
        frame True {
        }
      }
      n163 = call <vilib>:"CTRE_Phoenix_MotorControl_RefNumRegistryGet.vi"("refnum name"="Shooter") -> ("PhoenixMotorControlDevRef"=w153:T3)  [unwired: 9 in, 1 out]
      n164 = call <vilib>:"CTRE_Phoenix_MotorControl_RefNumRegistryGet.vi"("refnum name"="Hood Shooter") -> ("PhoenixMotorControlDevRef"=w150:T3)  [unwired: 9 in, 1 out]
      n165 = while {
        tunnel: w153 -> [w205]
        stop <- FALSE stop-if-true
        w226 = T18 2 items=["PercentOutput"=0, "Position"=1, "Velocity"=2, "Current"=3, "Follower"=5, "MotionProfile"=6, "MotionMagic"=7, "MotionProfileArc"=10, "Disabled"=15] ("Control Mode")
        w228 = T23 0 items=["QuadEncoder"=0, "Analog"=2, "Tachometer"=4, "Pulse Width Encoded Position"=8, "Sensor Sum (S0 + S1)"=9, "Sensor Difference (D0 - D1)"=10, "Remote Source 0"=11, "Remote Source 1"=12, "Software Emulated"=15] ("Feedback Device")
        # "Converts RPM to Sensor Units"
        # "Shooter PID Loop"
        n166 = global read "StateMachine_Global.vi" "Shooter Setpoint"() -> (w207:dbl)
        n167 = call <vilib>:"CTRE_Phoenix_MotorControl_ConfigClosedLoopRamp.vi"("secondsFromNeutralToFull"="Neutral to Full Seconds", "PhoenixMotorControlDevRef"=w205) -> ("error out"=w230:errorcluster, "PhoenixMotorControlDevRef"=w231:T3)  [unwired: 8 in]
        n168 = call <vilib>:"CTRE_Phoenix_MotorControl_ConfigSelectedFeedbackSensor_Enhanced.vi"("error in (no error)"=w230, "Feedback Device"=w228, "PhoenixMotorControlDevRef"=w231) -> ("PhoenixMotorControlDevRef"=w227:T3)  [unwired: 7 in, 1 out]
        n169 = call <vilib>:"CTRE_Phoenix_MotorControl_ConfigClosedLoopConstants.vi"("PhoenixMotorControlDevRef"=w227, "slotIdx"=0, "P"="P", "I"="I", "D"="D", "F"="kF", "I Zone"="I Zone") -> ("PhoenixMotorControlDevRef"=w218:T3)  [unwired: 7 in, 1 out]
        n170 = Divide(x=w207, y=600.0 ("x")) -> (x/y=w210:dbl)
        n171 = Multiply(x=w210, y=4096.0) -> (x*y=w208:dbl)
        n172 = call <vilib>:"CTRE_Phoenix_MotorControl_Set.vi"("Output"=w208, "Control Mode"=w226, "PhoenixMotorControlDevRef"=w218) -> ()  [unwired: 7 in, 2 out]
        n173 = call-poly <vilib>:"CTRE_Phoenix_MotorController_Get_Enhanced.vi"("PhoenixMotorControlDevRef"=w218) -> ("Percent Output"=w220:dbl)  [unwired: 10 in, 4 out]
        n174 = call-poly <vilib>:"CTRE_Phoenix_MotorController_Get_Enhanced.vi"("PhoenixMotorControlDevRef"=w218, "pidLoopIdx"=u32 0) -> ("Velocity (Raw Sensor Units per 100 ms)"=w214:i32)  [unwired: 10 in, 3 out]
        n175 = Bundle("Percent Output"=w220) -> (→"Voltage Chart":cluster{"Percent Output":dbl})  [unwired: 1 in]
        n176 = Divide(x=w214, y=4096.0) -> (x/y=w213:dbl)
        n177 = Multiply(x=600.0, y=w213) -> (x*y=w216:dbl)
        n178 = Bundle("Shooter Setpoint"=w207, w216) -> (→"Shooter PID Chart":cluster{"Shooter Setpoint":dbl, dbl})  [unwired: 1 in]
        n179 = Wait (ms)(milliseconds to wait=u32 20) -> ()  [unwired: 1 out]
      }
      n180 = while {
        tunnel: w150 -> [w174]
        stop <- FALSE stop-if-true
        w195 = T18 2 items=["PercentOutput"=0, "Position"=1, "Velocity"=2, "Current"=3, "Follower"=5, "MotionProfile"=6, "MotionMagic"=7, "MotionProfileArc"=10, "Disabled"=15] ("Control Mode")
        w198 = T23 0 items=["QuadEncoder"=0, "Analog"=2, "Tachometer"=4, "Pulse Width Encoded Position"=8, "Sensor Sum (S0 + S1)"=9, "Sensor Difference (D0 - D1)"=10, "Remote Source 0"=11, "Remote Source 1"=12, "Software Emulated"=15] ("Feedback Device")
        # "Converts RPM to Sensor Units"
        # "Hood Shooter PID Loop"
        n181 = global read "StateMachine_Global.vi" "Shooter Setpoint"() -> (w176:dbl)
        n182 = call <vilib>:"CTRE_Phoenix_MotorControl_ConfigClosedLoopRamp.vi"("secondsFromNeutralToFull"="Neutral to Full Seconds Hood", "PhoenixMotorControlDevRef"=w174) -> ("error out"=w200:errorcluster, "PhoenixMotorControlDevRef"=w201:T3)  [unwired: 8 in]
        n183 = call <vilib>:"CTRE_Phoenix_MotorControl_ConfigSelectedFeedbackSensor_Enhanced.vi"("error in (no error)"=w200, "Feedback Device"=w198, "PhoenixMotorControlDevRef"=w201) -> ("PhoenixMotorControlDevRef"=w197:T3)  [unwired: 7 in, 1 out]
        n184 = call <vilib>:"CTRE_Phoenix_MotorControl_ConfigClosedLoopConstants.vi"("PhoenixMotorControlDevRef"=w197, "slotIdx"=0, "P"="P Hood", "I"="I Hood", "D"="D Hood", "F"="kF Hood", "I Zone"="I Zone Hood") -> ("PhoenixMotorControlDevRef"=w187:T3)  [unwired: 7 in, 1 out]
        n185 = Divide(x=w176, y=600.0 ("x")) -> (x/y=w179:dbl)
        n186 = Multiply(x=w179, y=4096.0) -> (x*y=w177:dbl)
        n187 = call <vilib>:"CTRE_Phoenix_MotorControl_Set.vi"("Output"=w177, "Control Mode"=w195, "PhoenixMotorControlDevRef"=w187) -> ()  [unwired: 7 in, 2 out]
        n188 = call-poly <vilib>:"CTRE_Phoenix_MotorController_Get_Enhanced.vi"("PhoenixMotorControlDevRef"=w187) -> ("Percent Output"=w189:dbl)  [unwired: 10 in, 4 out]
        n189 = call-poly <vilib>:"CTRE_Phoenix_MotorController_Get_Enhanced.vi"("PhoenixMotorControlDevRef"=w187, "pidLoopIdx"=u32 0) -> ("Velocity (Raw Sensor Units per 100 ms)"=w183:i32)  [unwired: 10 in, 3 out]
        n190 = Bundle("Percent Output"=w189) -> (→"Voltage Chart Hood":cluster{"Percent Output":dbl})  [unwired: 1 in]
        n191 = Divide(x=w183, y=4096.0) -> (x/y=w182:dbl)
        n192 = Multiply(x=600.0, y=w182) -> (x*y=w185:dbl)
        n193 = Bundle("Shooter Setpoint"=w176, w185) -> (→"Shooter PID Chart Hood":cluster{"Shooter Setpoint":dbl, dbl})  [unwired: 1 in]
        n194 = Wait (ms)(milliseconds to wait=u32 20) -> ()  [unwired: 1 out]
      }
      n195 = while {
        stop <- FALSE stop-if-true
        # "Turret PID Loop"
        n196 = global read "StateMachine_Global.vi" "Turret Free Mode"() -> (w391:bool)
        n197 = global read "StateMachine_Global.vi" "Turret Setpoint"() -> (w389:dbl)
        n198 = global read "StateMachine_Global.vi" "Encoder?"() -> (w390:bool)
        n199 = case shown="False" w391 {
          tunnel: w390 -> [w401 _]
          tunnel: w389 -> [w399 _]
          tunnel: [w394 w406] -> w388
          tunnel: "TARange" -> [w398 _]
          tunnel: "TAIntegral Range" -> [w397 _]
          tunnel: "TADisable Range" -> [w396 _]
          tunnel: "TAGains" -> [w395 _]
          tunnel: [w394 _] -> w382
          tunnel: [w393 _] -> w381
          frame False {
            n200 = case shown="True" w401 {
              tunnel: [w403 w405] -> w400
              tunnel: [w402 w404] -> w393
              tunnel: w399 -> [w402 w404]
              frame False {
                n201 = global read "Actuators_n_Sensor_Global.vi" "LL X"() -> (w403:dbl)
              }
              frame True {
                n202 = global read "Actuators_n_Sensor_Global.vi" "TurretDegrees"() -> (w405:dbl)
              }
            }
            n203 = call "TurretAnglePID.vi"("TAGains"=w395, "TARange"=w398, "TADisable Range"=w396, "TAIntegral Range"=w397, "TAProcess variable"=w400, "TASetpoint"=w393) -> ("TAoutput"=w394:dbl)  [unwired: 5 in]
          }
          frame True {
            n204 = global read "Axes_n_Buttons_Global.vi" "OpAxis4"() -> (w408:dbl)
            n205 = Multiply(x=w408, y=0.4) -> (x*y=w406:dbl)
          }
        }
        n206 = global write "Actuators_n_Sensor_Global.vi" "TurretOutput"(w388) -> ()
        n207 = Bundle("Turret Setpoint"=w381, "TAoutput"=w382) -> (→"Turret PID Chart":cluster{"Turret Setpoint":dbl, "TAoutput":dbl})  [unwired: 1 in]
        n208 = Wait (ms)(milliseconds to wait=u32 20) -> ()  [unwired: 1 out]
      }
      n209 = while {
        stop <- FALSE stop-if-true
        # "Hood PID Loop"
        n210 = global read "StateMachine_Global.vi" "Hood Setpoint"() -> (w154:dbl)
        n211 = call "HoodPID.vi"("TASetpoint"=w154) -> ("TAoutput"=w156:dbl)  [unwired: 10 in]
        n212 = global write "Actuators_n_Sensor_Global.vi" "HoodOutput"(w156) -> ()
        n213 = Bundle("Hood Setpoint"=w154, "TAoutput"=w156) -> (→"Hood PID Chart":cluster{"Hood Setpoint":dbl, "TAoutput":dbl})  [unwired: 1 in]
        n214 = Wait (ms)(milliseconds to wait=u32 20) -> ()  [unwired: 1 out]
      }
    }
    frame Enabled {
    }
  }
  n215 = call <vilib>:"WPI_RobotDriveRefNum Registry Get.vi"("refnum name"="Drivetrain") -> ("RobotDriveDevRef"=w2:T14)  [unwired: 9 in, 1 out]
  n216 = while {
    tunnel: w2 -> [w418]
    stop <- FALSE stop-if-true
    # "Drivetrain Subsystem"
    n217 = disable-structure shown="Disabled" {
      disable-tunnel: [w424 _] -> _
      disable-tunnel: [w423 _] -> _
      frame Disabled {
        n218 = global read "Axes_n_Buttons_Global.vi" "DrAxis1"() -> (w424:dbl)
        n219 = global read "Axes_n_Buttons_Global.vi" "DrAxis4"() -> (w423:dbl)
      }
      frame Enabled {
      }
    }
    n220 = global read "Robot Global Data.vi" "Robot Mode"() -> (w422:T24)
    n221 = global read "StateMachine_Global.vi" "ClimberPull"() -> (w419:bool)
    n222 = Not Equal?(x=w422, y=WPI_DriverStationRobotMode2."Autonomous Enabled") -> (x != y?=w420:bool)
    n223 = case shown="True" w420 {
      tunnel: [w426 w442] -> w415
      tunnel: [w425 w441] -> w414
      tunnel: w419 -> [_ w435]
      frame False {
        n224 = global read "Axes_n_Buttons_Global.vi" "AutoRight"() -> (w425:dbl)
        n225 = global read "Axes_n_Buttons_Global.vi" "AutoLeft"() -> (w426:dbl)
      }
      frame True {
        n226 = case shown="False" w435 {
          tunnel: ["Sensitivity" 1.0 ("Sensitivity")] -> w432
          tunnel: [w450 0.0 ("DrAxis4")] -> w433
          tunnel: [w457 w463] -> w434
          tunnel: [w452 FALSE ("DrButton4")] -> w427
          tunnel: [w456 FALSE ("DrButton5")] -> w437
          tunnel: [w451 FALSE] -> w428
          frame False {
            # "Driver Control"
            n227 = global read "Axes_n_Buttons_Global.vi" "DrAxis1"() -> (w457:dbl)
            n228 = global read "Axes_n_Buttons_Global.vi" "DrAxis4"() -> (w458:dbl)
            n229 = global read "Axes_n_Buttons_Global.vi" "DrButton4"() -> (w453:bool)
            n230 = global read "Axes_n_Buttons_Global.vi" "DrAxis3"() -> (w455:dbl)
            n231 = global read "Axes_n_Buttons_Global.vi" "DrButton5"() -> (w456:bool)
            n232 = Greater Or Equal?(x=w455, y=0.75) -> (x >= y?=w451:bool)
            n233 = Negate(x=w458) -> (-x=w450:dbl)
            n234 = call "Toggle.vi"("In"=w453) -> ("Toggled"=w452:bool)  [unwired: 10 in]
          }
          frame True {
            # "Driver Control"
            n235 = global read "StateMachine_Global.vi" "ClimberOutput"() -> (w463:dbl)
          }
        }
        "Reversed?" <- w427
        n236 = case shown="True" w427 {
          tunnel: w434 -> [w445 w449]
          tunnel: w433 -> [w444 w447]
          tunnel: w432 -> [w443 w446]
          tunnel: [w445 w448] -> w431
          tunnel: [w444 w447] -> w430
          tunnel: [w443 w446] -> w429
          frame False {
            # "Default"
          }
          frame True {
            # "Reverse"
            n237 = Negate(x=w449) -> (-x=w448:dbl)
          }
        }
        n238 = case shown="True" w428 {
          tunnel: [w468 w473] -> w440
          tunnel: w429 -> [w468 w473]
          tunnel: [w466 w472] -> w439
          tunnel: w430 -> [w466 w471]
          tunnel: w431 -> [w467 w470]
          tunnel: [w467 w469] -> w438
          frame False {
            # "100% Output"
          }
          frame True {
            # "60% Output"
            n239 = call "60percent.vi"("In"=w470) -> ("Out"=w469:dbl)  [unwired: 10 in]
            n240 = call "60percent.vi"("In"=w471) -> ("Out"=w472:dbl)  [unwired: 10 in]
          }
        }
        n241 = call "CheesyDrive.vi"("Quickturn"=w437, "WheelNonLinearity"=0.65, "Sensitivty"=w440, "Wheel"=w439, "Throttle"=w438) -> ("Right PWM"=w441:dbl, "Left PWM"=w442:dbl)  [unwired: 5 in]
      }
    }
    n242 = call <vilib>:"WPI_RobotDriveTankDrive.vi"("Right axis value"=w414, "Left axis value"=w415, "RobotDriveDevRef"=w418) -> ()  [unwired: 6 in, 3 out]
    n243 = Wait (ms)(milliseconds to wait=u32 50) -> ()  [unwired: 1 out]
  }
  n244 = call "HoodPID.vi"() -> ()  [unwired: 11 in, 1 out]
